vi "Init.vi"(8 "error in (no error)":errorcluster, 11 "Config.lvlib:_ConfigClass_ApplSett_IN":refnum<class "_ConfigClass_INI.lvclass">) -> (0 "error out":errorcluster, 3 "Config.lvlib:_ConfigClass_ApplSett_OUT":refnum<class "_ConfigClass_INI.lvclass">)   [LabVIEW 2019, in "_ConfigClass_INI.lvlib" / "_ConfigClass_INI.lvclass"]
uses:
  _ConfigClass_INI.lvclass
  _ConfigClass_INI.lvclass/_ConfigClass_INI.ctl
  <vilib>/Utility/config.llb/NI_LVConfig.lvlib
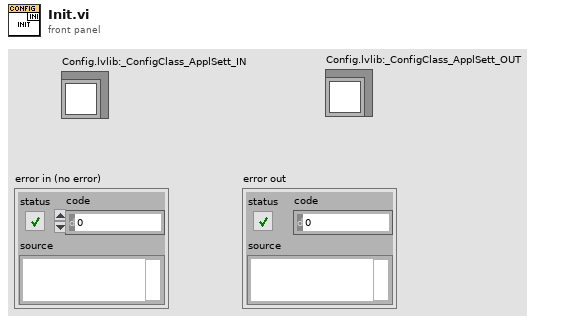
[diagram p1: front panel]
types:
  T1 = typedef "NI_LVConfig.lvlib/Config Data RefNum.ctl" = refnum<k1>
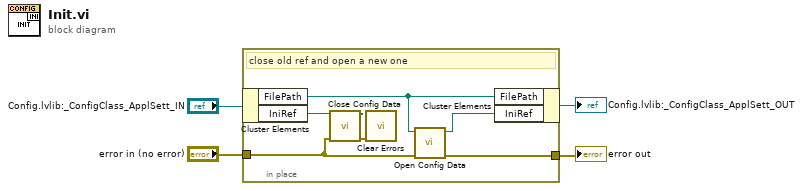
[diagram p0: block diagram]
diagram:
  n1 = in-place {
    in-place-border: "error in (no error)" -> [w6]
    in-place-border: [w10] -> w2
    # "close old ref and open a new one"
    n2 = in-place-cluster #1("Config.lvlib:_ConfigClass_ApplSett_IN") -> ("FilePath"=w9:path, "IniRef"=w7:T1)
    n3 = call <vilib>:"Close Config Data.vi"("error in (no error)"=w6, "refnum"=w7) -> ("error out"=w5:errorcluster)  [unwired: 8 in, 1 out]
    n4 = call <vilib>:"Clear Errors.vi"("error in (no error)"=w5) -> ()  [unwired: 5 in, 2 out]
    n5 = call <vilib>:"Open Config Data.vi"("error in (no error)"=w6, "configuration file path"=w9) -> ("error out"=w10:errorcluster, "refnum"=w8:T1)  [unwired: 7 in, 1 out]
    n6 = in-place-cluster #1("FilePath"=w9, "IniRef"=w8) -> (→"Config.lvlib:_ConfigClass_ApplSett_OUT":refnum<class "_ConfigClass_INI.lvclass">)
  }
  "error out" <- w2
